vi "lab1.vi"() -> ()   [LabVIEW 2023]
panel:
  in  "write buffer 4":string
  in  "write buffer 3":string
  in  "write buffer 2":string
  in  "write buffer":string
  in  "Write":bool
  in  "Exit":bool
  in  "Connect":bool
  in  "VISA resource name":refnum<visa-resource-name>
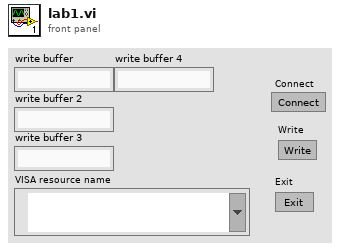
[diagram p1: front panel]
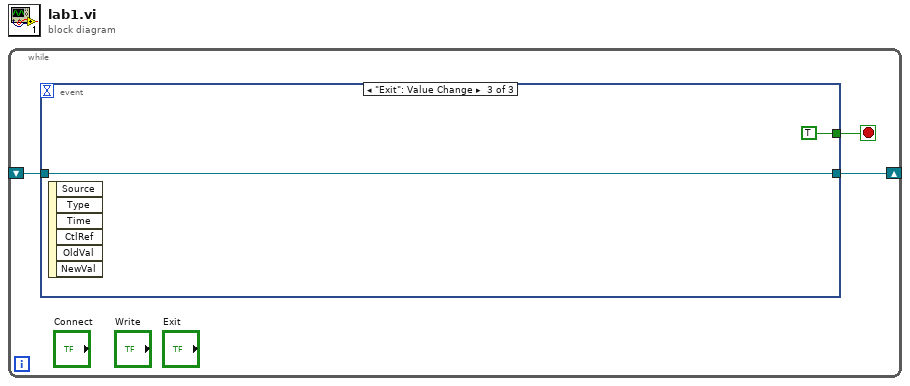
[diagram p0: block diagram]
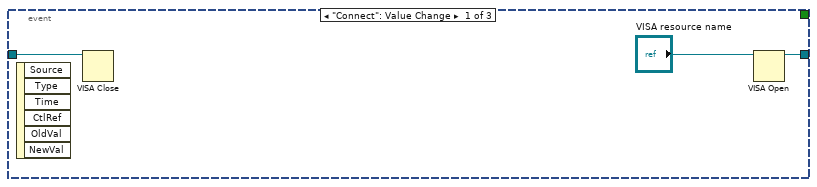
[diagram p2: hidden frame]
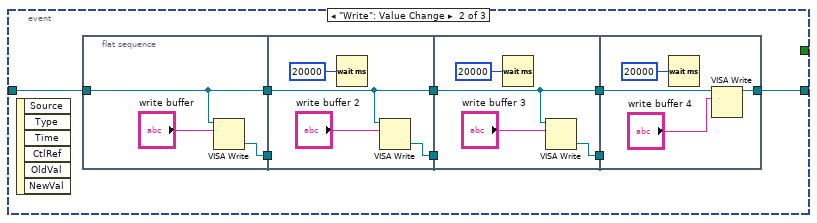
[diagram p3: hidden frame]
diagram:
  n1 = while {
    shift-right: [w1] -> _
    shift-left: _ -> [w3]
    stop <- w2 stop-if-true
    n2 = event shown="[2] \"Exit\": Value Change" {
      selector: _ -> [_ _ _]
      dyn-events: _ -> [_ _ _]
      timeout: _ -> [_ _ _]
      tunnel: [w4 w14 w30] -> w1
      tunnel: w3 -> [w5 w13 w30]
      tunnel: [_ _ TRUE] -> w2
      event "Connect": Value Change {
        n3 = event-data() -> ()  [unwired: 1 in, 6 out]
        n4 = VISA Close(VISA resource name=w5) -> ()  [unwired: 1 in, 1 out]
        n5 = VISA Open(VISA resource name="VISA resource name") -> (VISA resource name=w4:refnum<visa-resource-name>)  [unwired: 4 in, 1 out]
      }
      event "Write": Value Change {
        n6 = event-data() -> ()  [unwired: 1 in, 6 out]
        n7 = flat-sequence {
          tunnel: w13 -> [w17]
          tunnel: [w17] -> w12
          tunnel: [w16] -> w11
          tunnel: [w20] -> w10
          tunnel: [w19] -> w9
          tunnel: w12 -> [w20]
          tunnel: w11 -> [_]
          tunnel: w10 -> [w25]
          tunnel: [w25] -> w8
          tunnel: w9 -> [_]
          tunnel: [w24] -> w7
          tunnel: w8 -> [w29]
          tunnel: [w28] -> w14
          tunnel: w7 -> [_]
          frame #0 {
            n8 = VISA Write(VISA resource name=w17, write buffer="write buffer") -> (VISA resource name out=w16:refnum<visa-resource-name>)  [unwired: 1 in, 2 out]
          }
          frame #1 {
            n9 = Wait (ms)(milliseconds to wait=u32 20000) -> ()  [unwired: 1 out]
            n10 = VISA Write(VISA resource name=w20, write buffer="write buffer 2") -> (VISA resource name out=w19:refnum<visa-resource-name>)  [unwired: 1 in, 2 out]
          }
          frame #2 {
            n11 = Wait (ms)(milliseconds to wait=u32 20000) -> ()  [unwired: 1 out]
            n12 = VISA Write(VISA resource name=w25, write buffer="write buffer 3") -> (VISA resource name out=w24:refnum<visa-resource-name>)  [unwired: 1 in, 2 out]
          }
          frame #3 {
            n13 = Wait (ms)(milliseconds to wait=u32 20000) -> ()  [unwired: 1 out]
            n14 = VISA Write(VISA resource name=w29, write buffer="write buffer 4") -> (VISA resource name out=w28:refnum<visa-resource-name>)  [unwired: 1 in, 2 out]
          }
        }
      }
      event "Exit": Value Change {
        n15 = event-data() -> ()  [unwired: 1 in, 6 out]
      }
    }
  }
